vi "HAPS_main_Phase_Cali.vi"() -> ()   [LabVIEW 2023, in "HAPS.lvlib"]
uses:
  HAPS.lvlib
  MCU_Function.ctl
  set_ele.ctl
  HAPS_SerialPort.ctl
  HAPS_MCU_ELE_Func.ctl
panel:
  out "ele_gain":i32
  out "comn_gain":i32
  out "Duration":dbl
  in  "Init?":bool
  out "In-Phase : Phase(degree)":dbl[](graph)
  out "In-Phase : Gain(dB)":dbl[](graph)
  out "channel":i32
  out "chain_id":i32
  out "group":i32
  out "array_id":i32
  in  "Phase diff. Criteria":dbl format="%#_13g"
  in  "Tx/Rx":enum16{"Rx", "Tx"}(ring)=enum."Tx"
  in  "array_id (MCU index)":i32
  in  "MCU_UART_addr":refnum<visa-resource-name>="COM1"
  in  "Max Steps":i32=10
  in  "Target(degree)":dbl format="%#_13g"
  in  "SweepPoints":i32=11
  in  "sParameter":i32=21
  in  "Stop_Freq(GHz)":dbl=39.5
  in  "Start_Freq(GHz)":dbl=38.5
  in  "VISA resource name":refnum<visa-resource-name>="TCPIP0::192.168.119.45::inst0::INSTR"
  in  "HAPS_Equipment":enum16{"Keysight", "R&S"}(ring)=enum."R&S"
  # "TCPIP0::192.168.119.45::inst0::INSTR"
  # "HAPS_24x24_Phase_Calibration"
  # "VNA"
  # "TCPIP0::192.168.1.31::hislip0::INSTR"
  # "Test Status"
  # "DUT"
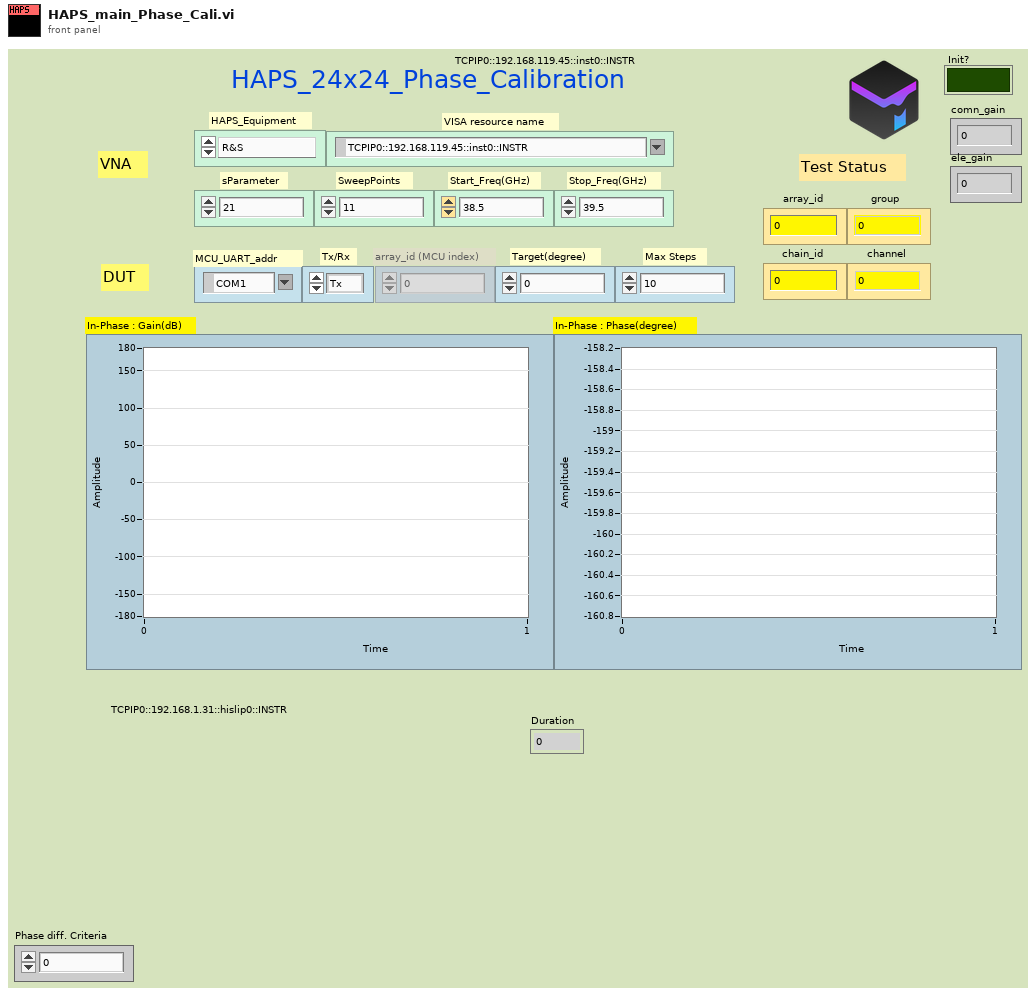
[diagram p1: front panel]
types:
  T1 = typedef "HAPS.lvlib/HAPS_SerialPort.ctl" = enum16{"Init", "Close", "CMD", "Flush"}
  T2 = typedef "HAPS.lvlib/HAPS_MCU_ELE_Func.ctl" = enum16{"array_init", "set_com_gain", "set_ch_gain_phase", "set_pd_range", "get_preamp_temp", "get_bfic_temp", "get_tx_pd", "ch_on", "ch_on_2", "ch_ctrl_all", "array_ctrl_src"}
  T3 = typedef "HAPS.lvlib/set_ele.ctl" = cluster{"ch":i32, "chain_id":i32, "group":i32, "array_id":i32, "ele_phase":i32, "ele_gain":i32, "com_gain":i32, "pd_range":i32}
  T4 = typedef "HAPS.lvlib/MCU_Function.ctl" = cluster{"Tx/Rx":enum16{"Rx", "Tx"}, "Enable?":enum16{"OFF", "On"}, "Source":enum16{"MCU", "ACU"}}
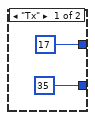
[diagram p2: hidden frame]
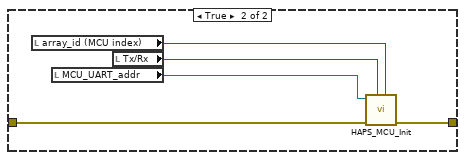
[diagram p3: hidden frame]
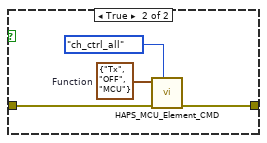
[diagram p4: hidden frame]
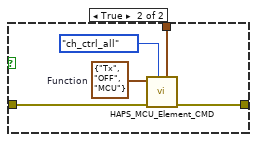
[diagram p6: hidden frame]
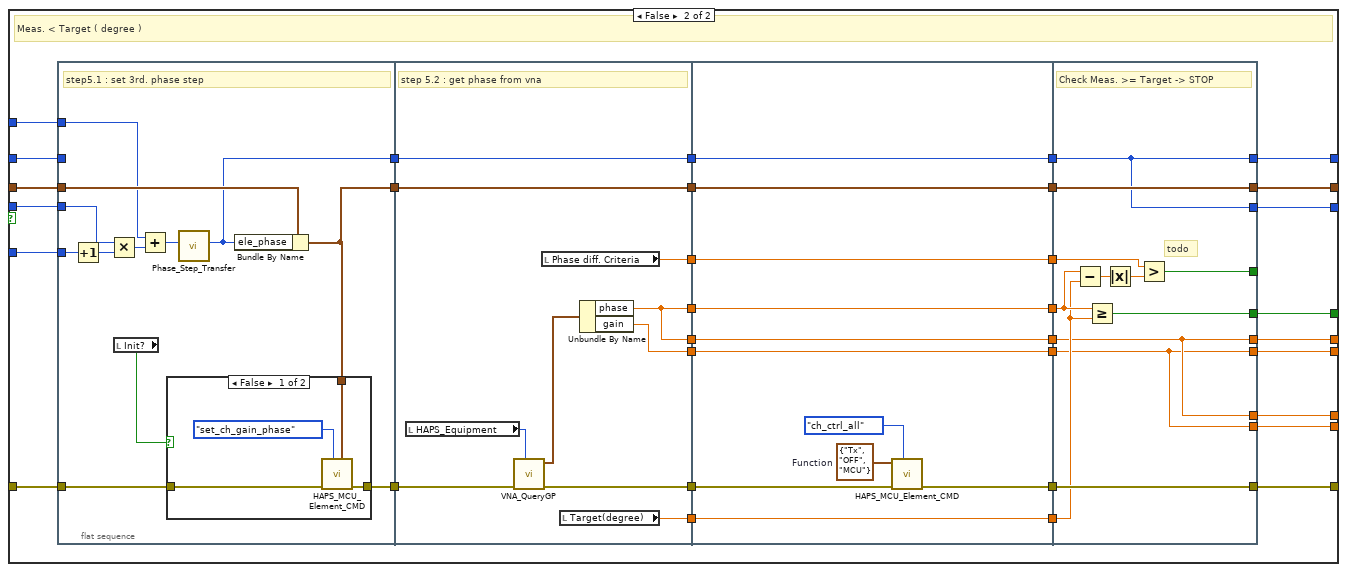
[diagram p10: hidden frame]
diagram:
  n1 = flat-sequence {
    tunnel: [w23] -> w16
    tunnel: [w30] -> w15
    tunnel: [errorcluster {"status"=FALSE, "code"=0, "source"=""} ("error in")] -> w13
    tunnel: ["sParameter"] -> w11
    tunnel: ["VISA resource name"] -> w10
    tunnel: ["Start_Freq(GHz)"] -> w9
    tunnel: ["Stop_Freq(GHz)"] -> w8
    tunnel: ["SweepPoints"] -> w7
    tunnel: ["HAPS_Equipment"] -> w6
    tunnel: [w20] -> w4
    tunnel: w16 -> [w47]
    tunnel: w15 -> [_]
    tunnel: [w47] -> w14
    tunnel: w13 -> [w46]
    tunnel: [w38] -> w12
    tunnel: w11 -> [w45]
    tunnel: w10 -> [w44]
    tunnel: w9 -> [w43]
    tunnel: w8 -> [w42]
    tunnel: w7 -> [w41]
    tunnel: w6 -> [w37]
    tunnel: [w35] -> w5
    tunnel: w4 -> [w35]
    tunnel: w14 -> [w66]
    tunnel: w12 -> [w67]
    tunnel: w5 -> [w63]
    tunnel: [w63] -> w3
    tunnel: [w62] -> w2
    tunnel: [w60] -> w1
    tunnel: [w509] -> _
    tunnel: w3 -> [w509]
    tunnel: w2 -> [w511]
    tunnel: w1 -> [w501]
    frame #0 {
      w21 = dbl[] []
      w23 = T3 {"ch"=0, "chain_id"=0, "group"=0, "array_id"=0, "ele_phase"=0, "ele_gain"=0, "com_gain"=0, "pd_range"=0}  # set_ele
      w30 = T4 {"Tx/Rx"=enum."Tx", "Enable?"=enum."OFF", "Source"=enum."MCU"}  # Function
      # "Init"
      n2 = case shown="\"Rx\"" "Tx/Rx" {
        tunnel: [17 ("comn_ele_gain") 17 ("comn_ele_gain")] -> w18
        tunnel: [35 ("comn_ele_gain") 22 ("comn_ele_gain")] -> w17
        frame "Tx" {
        }
        frame "Rx" {
        }
      }
      "comn_gain" <- w18
      "ele_gain" <- w17
      n3 = Get Date/Time In Seconds() -> (seconds since 1Jan1904=w20:timestamp)
      "In-Phase : Gain(dB)" <- w21
      "In-Phase : Phase(degree)" <- w21
    }
    frame #1 {
      # "settting before Calibration"
      n4 = call "VNA_init.vi"("Stop_Freq(GHz)"=w42, "HAPS_MCU_CMD"=w37, "Start_Freq(GHz)"=w43, "sParameter"=w45, "error in"=w46, "SweepPoints"=w41, "Mark no."=1, "VISA resource name"=w44) -> ("error out"=w39:errorcluster)  [unwired: 3 in]
      n5 = case shown="False" "Init?" {
        tunnel: w39 -> [w54 w59]
        tunnel: [w50 w58] -> w38
        frame False {
          n6 = local read "MCU_UART_addr"() -> (w52:refnum<visa-resource-name>)
          n7 = call "HAPS_MCU_SerialPort.vi"("HAPS_SerialPort_Func"=HAPS_SerialPort."Init", "error in"=w54, "VISA resource name"=w52) -> ("error out"=w51:errorcluster)  [unwired: 6 in, 2 out]
          n8 = call "HAPS_MCU_SerialPort.vi"("Command"="log_en 0", "HAPS_SerialPort_Func"=enum16{"Init", "Close", "CMD"}."CMD" ("HAPS_SerialPort"), "error in"=w51) -> ("error out"=w50:errorcluster)  [unwired: 6 in, 2 out]
        }
        frame True {
          n9 = local read "array_id (MCU index)"() -> (w56:i32)
          n10 = local read "MCU_UART_addr"() -> (w57:refnum<visa-resource-name>)
          n11 = local read "Tx/Rx"() -> (w55:enum16{"Rx", "Tx"})
          n12 = call "HAPS_MCU_Init.vi"("array_id"=w56, "Tx/Rx"=w55, "error in"=w59, "VISA resource name"=w57) -> ("error out"=w58:errorcluster)  [unwired: 7 in]
        }
      }
    }
    frame #2 {
      # "Calibration"
      n13 = for {
        N: 1 -> [_]
        shift-right: [w77] -> _
        shift-left: w66 -> [w73]
        shift-right: [w76] -> w62
        shift-left: string[][] [] -> [w71]
        shift-right: [w75] -> _
        shift-left: w67 -> [w74]
        shift-right: [w68] -> w60
        shift-left: string[][] [] -> [w69]
        i -> [w72]
        w70 = dbl[] []
        # "group ( 0~2 )"
        n14 = for {
          N: 1 -> [_]
          shift-right: [w92] -> w77
          shift-left: w73 -> [w88]
          shift-right: [w91] -> w76
          shift-left: w71 -> [w85]
          shift-right: [w90] -> w75
          shift-left: w74 -> [w89]
          tunnel: w72 -> [w87]
          shift-right: [w82] -> _
          shift-left: w70 -> [w84]
          shift-right: [w81] -> _
          shift-left: w70 -> [w83]
          shift-right: [w79] -> w68
          shift-left: w69 -> [w80]
          i -> [w86]
          # "Chain_id ( 0~11 )"
          n15 = for {
            N: 2 -> [_]
            shift-right: [w164] -> w92
            shift-left: w88 -> [w98]
            shift-right: [w154] -> w91
            shift-left: w85 -> [w155]
            shift-right: [w96] -> w90
            shift-left: w89 -> [w104]
            tunnel: w87 -> [w101]
            tunnel: w86 -> [w100]
            shift-right: [w144] -> w82
            shift-left: w84 -> [w151]
            shift-right: [w143] -> w81
            shift-left: w83 -> [w149]
            shift-right: [w138] -> w79
            shift-left: w80 -> [w142]
            i -> [w99]
            # "Channel ( 0~15 )"
            n16 = local read "array_id (MCU index)"() -> (w102:i32)
            n17 = Bundle By Name(cluster=w98, "array_id"=w102, "group"=w101, "chain_id"=w100, "ch"=w99) -> (w97:T3)
            n18 = call "HAPS_MCU_Element_CMD.vi"("set_ele"=w97, "HAPS_MCU_ELE_Func."=HAPS_MCU_ELE_Func."ch_on", "error in"=w104) -> ("error out"=w103:errorcluster)  [unwired: 7 in, 1 out]
            n19 = flat-sequence {
              tunnel: w97 -> [w188]
              tunnel: w103 -> [w189]
              tunnel: [w190] -> w169
              tunnel: [w186] -> w167
              tunnel: w99 -> [w185]
              tunnel: [w184] -> w156
              tunnel: w155 -> [w184]
              tunnel: w101 -> [w182]
              tunnel: w100 -> [w181]
              tunnel: [w180] -> w152
              tunnel: w151 -> [w180]
              tunnel: [w179] -> w150
              tunnel: w149 -> [w179]
              tunnel: w142 -> [w178]
              tunnel: [w178] -> w141
              tunnel: w169 -> [w206]
              tunnel: [w207] -> w137
              tunnel: [w205] -> w135
              tunnel: [w204] -> w133
              tunnel: w167 -> [w204]
              tunnel: [w201] -> w131
              tunnel: w156 -> [w201]
              tunnel: [w200] -> w129
              tunnel: w152 -> [w200]
              tunnel: [w199] -> w127
              tunnel: w150 -> [w199]
              tunnel: w141 -> [w198]
              tunnel: [w198] -> w125
              tunnel: w137 -> [w213]
              tunnel: [w214] -> w136
              tunnel: w135 -> [w219]
              tunnel: [w219] -> w134
              tunnel: w133 -> [w212]
              tunnel: [w212] -> w132
              tunnel: w131 -> [w218]
              tunnel: [w218] -> w130
              tunnel: w129 -> [w217]
              tunnel: [w217] -> w128
              tunnel: w127 -> [w216]
              tunnel: [w216] -> w126
              tunnel: w125 -> [w215]
              tunnel: [w215] -> w124
              tunnel: w136 -> [w234]
              tunnel: w134 -> [w231]
              tunnel: w132 -> [w233]
              tunnel: [w235] -> w168
              tunnel: [w232] -> w166
              tunnel: [w231] -> w165
              tunnel: [w230] -> w157
              tunnel: w130 -> [w230]
              tunnel: w128 -> [w229]
              tunnel: w126 -> [w228]
              tunnel: [w229] -> w148
              tunnel: [w228] -> w147
              tunnel: w124 -> [w227]
              tunnel: [w227] -> w140
              tunnel: w168 -> [w255]
              tunnel: w166 -> [w247]
              tunnel: [w256] -> w123
              tunnel: [w250] -> w121
              tunnel: [w249] -> w119
              tunnel: [w247] -> w117
              tunnel: [w246] -> w115
              tunnel: w165 -> [w246]
              tunnel: [w244] -> w113
              tunnel: w157 -> [w244]
              tunnel: [w243] -> w111
              tunnel: w148 -> [w243]
              tunnel: [w242] -> w109
              tunnel: w147 -> [w242]
              tunnel: w140 -> [w241]
              tunnel: [w241] -> w107
              tunnel: w123 -> [w258]
              tunnel: [w259] -> w122
              tunnel: w121 -> [w267]
              tunnel: [w267] -> w120
              tunnel: w119 -> [w266]
              tunnel: [w266] -> w118
              tunnel: w117 -> [w265]
              tunnel: [w265] -> w116
              tunnel: w115 -> [w264]
              tunnel: [w264] -> w114
              tunnel: w113 -> [w263]
              tunnel: [w263] -> w112
              tunnel: w111 -> [w262]
              tunnel: [w262] -> w110
              tunnel: w109 -> [w261]
              tunnel: [w261] -> w108
              tunnel: w107 -> [w260]
              tunnel: [w260] -> w106
              tunnel: w122 -> [w285]
              tunnel: w120 -> [w286]
              tunnel: w118 -> [w287]
              tunnel: w116 -> [w288]
              tunnel: w114 -> [w273]
              tunnel: [w284] -> w163
              tunnel: [w283] -> w162
              tunnel: [w282] -> w161
              tunnel: [w281] -> w160
              tunnel: [w280] -> w159
              tunnel: [w279] -> w158
              tunnel: w112 -> [w279]
              tunnel: [w278] -> w153
              tunnel: w110 -> [w277]
              tunnel: w108 -> [w276]
              tunnel: [w277] -> w146
              tunnel: [w276] -> w145
              tunnel: w106 -> [w275]
              tunnel: [w274] -> w139
              tunnel: [w500] -> w164
              tunnel: w163 -> [w500]
              tunnel: w162 -> [w499]
              tunnel: w161 -> [w471]
              tunnel: w160 -> [w472]
              tunnel: w159 -> [w494]
              tunnel: w158 -> [w478]
              tunnel: [w480] -> w154
              tunnel: [w479] -> w95
              tunnel: w153 -> [w479]
              tunnel: w146 -> [w475]
              tunnel: w145 -> [w474]
              tunnel: [w477] -> w144
              tunnel: [w476] -> w143
              tunnel: w139 -> [w470]
              tunnel: [w470] -> w138
              frame #0 {
                w191 = 0  # pd_range
                w192 = 0  # Init_Phase_Step
                # "step 1. : First get phase step \"0\" for element BFIC"
                n20 = local read "array_id (MCU index)"() -> (w183:i32)
                "array_id" <- w183
                n21 = local read "ele_gain"() -> (w175:i32)
                n22 = local read "comn_gain"() -> (w176:i32)
                n23 = Bundle By Name(cluster=w188, "array_id"=w183, "group"=w182, "chain_id"=w181, "ch"=w185, "com_gain"=w176, "ele_gain"=w175, "ele_phase"=w192, "pd_range"=w191) -> (w186:T3)
                n24 = case shown="False" FALSE {
                  tunnel: [w196 w197] -> w190
                  tunnel: w189 -> [w195 w197]
                  tunnel: HAPS_MCU_ELE_Func."set_ch_gain_phase" ("HAPS_MCU_ELE_Func.") -> [w194 _]
                  tunnel: w186 -> [w193 _]
                  frame False {
                    n25 = call "HAPS_MCU_Element_CMD.vi"("set_ele"=w193, "HAPS_MCU_ELE_Func."=w194, "error in"=w195) -> ("error out"=w196:errorcluster)  [unwired: 7 in, 1 out]
                  }
                  frame True {
                  }
                }
                "group" <- w182
                "chain_id" <- w181
                "channel" <- w185
              }
              frame #1 {
                # "todo:gain"
                # "step 2. : get first pahse data from vna"
                n26 = local read "HAPS_Equipment"() -> (w202:enum16{"Keysight", "R&S"})
                n27 = call "VNA_QueryGP.vi"("HAPS_Equipment"=w202, "error in"=w206) -> ("error out"=w207:errorcluster, "queryMarker"=w208:cluster{"gain":dbl, "phase":dbl})  [unwired: 8 in]
                n28 = Unbundle By Name(w204) -> ("ele_phase"=w203:i32)
                n29 = local read "Target(degree)"() -> (w210:dbl)
                n30 = Unbundle By Name(w208) -> ("phase"=w209:dbl)  [unwired: 1 out]
                n31 = call "Estimation_Steps.vi"("Target(degree)"=w210, "Source_Phase_Step"=w203, "Input_Phase(degree)"=w209) -> ("Esitmation_Step"=w205:i32)  [unwired: 7 in, 1 out]
              }
              frame #2 {
                n32 = case shown="False" FALSE {
                  tunnel: [w220 w225] -> w214
                  tunnel: w213 -> [w220 w224]
                  tunnel: w212 -> [_ w222]
                  frame False {
                  }
                  frame True {
                    w221 = T4 {"Tx/Rx"=enum."Tx", "Enable?"=enum."OFF", "Source"=enum."MCU"}  # Function
                    n33 = call "HAPS_MCU_Element_CMD.vi"("set_ele"=w222, "HAPS_MCU_ELE_Func."=HAPS_MCU_ELE_Func."ch_ctrl_all", "error in"=w224, "Function"=w221) -> ("error out"=w225:errorcluster)  [unwired: 6 in, 1 out]
                  }
                }
              }
              frame #3 {
                # "source.\nphase step"
                # "step 3.  set estimation phase step in second time"
                n34 = Bundle By Name(cluster=w233, "ele_phase"=w231) -> (w232:T3)
                n35 = case shown="False" FALSE {
                  tunnel: [w239 w240] -> w235
                  tunnel: w234 -> [w238 w240]
                  tunnel: w232 -> [w237 _]
                  frame False {
                    n36 = call "HAPS_MCU_Element_CMD.vi"("set_ele"=w237, "HAPS_MCU_ELE_Func."=HAPS_MCU_ELE_Func."set_ch_gain_phase", "error in"=w238) -> ("error out"=w239:errorcluster)  [unwired: 7 in, 1 out]
                  }
                  frame True {
                  }
                }
              }
              frame #4 {
                # "todo:gain"
                # "step 4. : get second time pahse from vna"
                n37 = local read "HAPS_Equipment"() -> (w245:enum16{"Keysight", "R&S"})
                n38 = call "VNA_QueryGP.vi"("HAPS_Equipment"=w245, "error in"=w255) -> ("error out"=w256:errorcluster, "queryMarker"=w251:cluster{"gain":dbl, "phase":dbl})  [unwired: 8 in]
                n39 = Unbundle By Name(w251) -> ("phase"=w248:dbl)  [unwired: 1 out]
                n40 = local read "Target(degree)"() -> (w252:dbl)
                n41 = Greater Or Equal?(x=w248, y=w252) -> (x >= y?=w250:bool)
                n42 = Select(t=1, s=w250, f=-1) -> (s? t:f=w249:i32)
              }
              frame #5 {
                n43 = local read "Init?"() -> (w257:bool)
                n44 = case shown="False" w257 {
                  tunnel: [w269 w272] -> w259
                  tunnel: w258 -> [w268 w272]
                  frame False {
                    w271 = T4 {"Tx/Rx"=enum."Tx", "Enable?"=enum."OFF", "Source"=enum."MCU"}  # Function
                    n45 = call "HAPS_MCU_Element_CMD.vi"("HAPS_MCU_ELE_Func."=HAPS_MCU_ELE_Func."ch_ctrl_all", "error in"=w268, "Function"=w271) -> ("error out"=w269:errorcluster)  [unwired: 7 in, 1 out]
                  }
                  frame True {
                  }
                }
              }
              frame #6 {
                # "source.\nphase step"
                # "Mea. >= Target"
                # "source.\ndegree"
                # "step 5. : find in-phase step"
                n46 = for {
                  N: "Max Steps" -> [_]
                  shift-right: [w313] -> w284
                  shift-left: w288 -> [w316]
                  shift-right: [w314] -> w278
                  shift-left: w285 -> [w319]
                  shift-right: [w307] -> w280
                  shift-left: w273 -> [w315]
                  tunnel: w286 -> [w320]
                  tunnel: w287 -> [w317]
                  shift-right: [w312] -> w283
                  shift-left: _ -> [_]
                  shift-right: [w298] -> w281
                  shift-left: _ -> [_]
                  shift-right: [w297] -> w282
                  shift-left: _ -> [_]
                  shift-right: [w291] -> w274
                  shift-left: w275 -> [w293]
                  tunnel: w273 -> [w290]
                  i -> [w318]
                  stop <- w312 stop-if-true
                  n47 = case shown="True" w320 {
                    tunnel: w319 -> [w346 w419]
                    tunnel: w318 -> [w345 w418]
                    tunnel: w317 -> [w344 w417]
                    tunnel: w316 -> [w343 w416]
                    tunnel: w315 -> [w342 w415]
                    tunnel: [w341 w414] -> w314
                    tunnel: [w340 w413] -> w313
                    tunnel: [w339 w412] -> w307
                    tunnel: [w331 w408] -> w312
                    tunnel: [w330 w407] -> _
                    tunnel: [w327 w406] -> w298
                    tunnel: [w326 w405] -> w297
                    tunnel: [w323 w404] -> _
                    tunnel: [w322 w403] -> _
                    tunnel: w290 -> [w321 w402]
                    frame True {
                      # "Meas. >= Target ( degree )"
                      n48 = flat-sequence {
                        tunnel: w346 -> [w355]
                        tunnel: w345 -> [w358]
                        tunnel: w344 -> [w357]
                        tunnel: w343 -> [w352]
                        tunnel: w342 -> [_]
                        tunnel: [w356] -> w338
                        tunnel: [w353] -> w337
                        tunnel: [w349] -> w336
                        tunnel: w321 -> [w347]
                        tunnel: w338 -> [w370]
                        tunnel: w337 -> [w373]
                        tunnel: w336 -> [w372]
                        tunnel: [w371] -> w335
                        tunnel: [w373] -> w334
                        tunnel: [w372] -> w333
                        tunnel: [w367] -> w332
                        tunnel: [w368] -> w329
                        tunnel: [w364] -> w328
                        tunnel: [w366] -> w325
                        tunnel: [w367] -> w324
                        tunnel: [w383] -> w331
                        tunnel: [w382] -> w339
                        tunnel: [w384] -> w340
                        tunnel: [w385] -> w341
                        tunnel: w335 -> [w385]
                        tunnel: w334 -> [w384]
                        tunnel: w333 -> [w382]
                        tunnel: w332 -> [w381]
                        tunnel: [w382] -> w330
                        tunnel: w329 -> [w379]
                        tunnel: w328 -> [w377]
                        tunnel: [w376] -> _
                        tunnel: [w375] -> w327
                        tunnel: [w374] -> w326
                        tunnel: w325 -> [w374]
                        tunnel: w324 -> [w375]
                        tunnel: [w375] -> w323
                        tunnel: [w374] -> w322
                        frame #0 {
                          # "step5.1 : set 3rd. phase step"
                          n49 = Increment(x=w358) -> (x+1=w354:i32)
                          n50 = local read "Init?"() -> (w348:bool)
                          n51 = Multiply(x=w357, y=w354) -> (x*y=w351:i32)
                          n52 = Add(x=w347, y=w351) -> (x+y=w350:i32)
                          n53 = call "Phase_Step_Transfer.vi"("Input_Phase_Step"=w350) -> ("Output_Phase_Step"=w349:i32)  [unwired: 10 in]
                          n54 = Bundle By Name(cluster=w352, "ele_phase"=w349) -> (w353:T3)
                          n55 = case shown="False" w348 {
                            tunnel: [w362 w363] -> w356
                            tunnel: w355 -> [w361 w363]
                            tunnel: w353 -> [w360 _]
                            frame False {
                              n56 = call "HAPS_MCU_Element_CMD.vi"("set_ele"=w360, "HAPS_MCU_ELE_Func."=HAPS_MCU_ELE_Func."set_ch_gain_phase", "error in"=w361) -> ("error out"=w362:errorcluster)  [unwired: 7 in, 1 out]
                            }
                            frame True {
                            }
                          }
                        }
                        frame #1 {
                          # "step 5.2 : get phase from vna"
                          n57 = local read "HAPS_Equipment"() -> (w365:enum16{"Keysight", "R&S"})
                          n58 = call "VNA_QueryGP.vi"("HAPS_Equipment"=w365, "error in"=w370) -> ("error out"=w371:errorcluster, "queryMarker"=w369:cluster{"gain":dbl, "phase":dbl})  [unwired: 8 in]
                          n59 = local read "Phase diff. Criteria"() -> (w364:dbl)
                          n60 = local read "Target(degree)"() -> (w368:dbl)
                          n61 = Unbundle By Name(w369) -> ("phase"=w367:dbl, "gain"=w366:dbl)
                        }
                        frame #2 {
                          # "todo"
                          # "Check Meas. <= Target => STOP"
                          n62 = Subtract(x=w381, y=w379) -> (x-y=w380:dbl)
                          n63 = Less Or Equal?(x=w381, y=w379) -> (x <= y?=w383:bool)
                          n64 = Absolute Value(x=w380) -> (abs(x)=w378:dbl)
                          n65 = Greater?(x=w377, y=w378) -> (0:w376:bool)
                        }
                      }
                    }
                    frame False {
                      # "Meas. < Target ( degree )"
                      n66 = flat-sequence {
                        tunnel: w419 -> [w428]
                        tunnel: w418 -> [w431]
                        tunnel: w417 -> [w430]
                        tunnel: w416 -> [w425]
                        tunnel: w415 -> [_]
                        tunnel: [w429] -> w411
                        tunnel: [w426] -> w410
                        tunnel: [w422] -> w409
                        tunnel: w402 -> [w420]
                        tunnel: w411 -> [w443]
                        tunnel: w410 -> [w446]
                        tunnel: w409 -> [w445]
                        tunnel: [w444] -> w401
                        tunnel: [w446] -> w399
                        tunnel: [w445] -> w397
                        tunnel: [w440] -> w395
                        tunnel: [w441] -> w393
                        tunnel: [w437] -> w391
                        tunnel: [w439] -> w389
                        tunnel: [w440] -> w387
                        tunnel: w401 -> [w447]
                        tunnel: [w448] -> w400
                        tunnel: w399 -> [w457]
                        tunnel: [w457] -> w398
                        tunnel: w397 -> [w456]
                        tunnel: [w456] -> w396
                        tunnel: w395 -> [w455]
                        tunnel: [w455] -> w394
                        tunnel: w393 -> [w454]
                        tunnel: [w454] -> w392
                        tunnel: w391 -> [w453]
                        tunnel: [w453] -> w390
                        tunnel: w389 -> [w452]
                        tunnel: [w452] -> w388
                        tunnel: w387 -> [w451]
                        tunnel: [w451] -> w386
                        tunnel: [w467] -> w408
                        tunnel: [w466] -> w412
                        tunnel: [w468] -> w413
                        tunnel: [w469] -> w414
                        tunnel: w400 -> [w469]
                        tunnel: w398 -> [w468]
                        tunnel: w396 -> [w466]
                        tunnel: w394 -> [w465]
                        tunnel: [w466] -> w407
                        tunnel: w392 -> [w463]
                        tunnel: w390 -> [w461]
                        tunnel: [w460] -> _
                        tunnel: [w459] -> w406
                        tunnel: [w458] -> w405
                        tunnel: w388 -> [w458]
                        tunnel: w386 -> [w459]
                        tunnel: [w459] -> w404
                        tunnel: [w458] -> w403
                        frame #0 {
                          # "step5.1 : set 3rd. phase step"
                          n67 = Increment(x=w431) -> (x+1=w427:i32)
                          n68 = Multiply(x=w430, y=w427) -> (x*y=w424:i32)
                          n69 = local read "Init?"() -> (w421:bool)
                          n70 = Add(x=w420, y=w424) -> (x+y=w423:i32)
                          n71 = call "Phase_Step_Transfer.vi"("Input_Phase_Step"=w423) -> ("Output_Phase_Step"=w422:i32)  [unwired: 10 in]
                          n72 = Bundle By Name(cluster=w425, "ele_phase"=w422) -> (w426:T3)
                          n73 = case shown="False" w421 {
                            tunnel: [w435 w436] -> w429
                            tunnel: w428 -> [w434 w436]
                            tunnel: w426 -> [w433 _]
                            frame False {
                              n74 = call "HAPS_MCU_Element_CMD.vi"("set_ele"=w433, "HAPS_MCU_ELE_Func."=HAPS_MCU_ELE_Func."set_ch_gain_phase", "error in"=w434) -> ("error out"=w435:errorcluster)  [unwired: 7 in, 1 out]
                            }
                            frame True {
                            }
                          }
                        }
                        frame #1 {
                          # "step 5.2 : get phase from vna"
                          n75 = local read "HAPS_Equipment"() -> (w438:enum16{"Keysight", "R&S"})
                          n76 = call "VNA_QueryGP.vi"("HAPS_Equipment"=w438, "error in"=w443) -> ("error out"=w444:errorcluster, "queryMarker"=w442:cluster{"gain":dbl, "phase":dbl})  [unwired: 8 in]
                          n77 = local read "Phase diff. Criteria"() -> (w437:dbl)
                          n78 = local read "Target(degree)"() -> (w441:dbl)
                          n79 = Unbundle By Name(w442) -> ("phase"=w440:dbl, "gain"=w439:dbl)
                        }
                        frame #2 {
                          w449 = T4 {"Tx/Rx"=enum."Tx", "Enable?"=enum."OFF", "Source"=enum."MCU"}  # Function
                          n80 = call "HAPS_MCU_Element_CMD.vi"("HAPS_MCU_ELE_Func."=HAPS_MCU_ELE_Func."ch_ctrl_all", "error in"=w447, "Function"=w449) -> ("error out"=w448:errorcluster)  [unwired: 7 in, 1 out]
                        }
                        frame #3 {
                          # "todo"
                          # "Check Meas. >= Target -> STOP"
                          n81 = Subtract(x=w465, y=w463) -> (x-y=w464:dbl)
                          n82 = Greater Or Equal?(x=w465, y=w463) -> (x >= y?=w467:bool)
                          n83 = Absolute Value(x=w464) -> (abs(x)=w462:dbl)
                          n84 = Greater?(x=w461, y=w462) -> (0:w460:bool)
                        }
                      }
                    }
                  }
                  n85 = property on="Tx/Rx" class="Enum (strict)"() -> ("RingText.Text"=w306:string)  [unwired: 2 in, 2 out]
                  n86 = local read "chain_id"() -> (w310:i32)
                  n87 = local read "array_id"() -> (w308:i32)
                  n88 = local read "channel"() -> (w311:i32)
                  n89 = local read "group"() -> (w309:i32)
                  n90 = Number To Decimal String(number=w308) -> (decimal integer string=w305:string)  [unwired: 1 in]
                  n91 = Number To Decimal String(number=w309) -> (decimal integer string=w304:string)  [unwired: 1 in]
                  n92 = Number To Decimal String(number=w310) -> (decimal integer string=w303:string)  [unwired: 1 in]
                  n93 = Number To Decimal String(number=w311) -> (decimal integer string=w302:string)  [unwired: 1 in]
                  n94 = Number To Decimal String(number=w307) -> (decimal integer string=w301:string)  [unwired: 1 in]
                  n95 = Number To Fractional String(number=w298, precision (6)=i16 3) -> (F-format string=w296:string)  [unwired: 2 in]
                  n96 = Number To Fractional String(number=w297, precision (6)=i16 3) -> (F-format string=w295:string)  [unwired: 2 in]
                  n97 = Build Array(w306, w305, w304, w303, w302, w301, w296, w295, "log") -> (w292:string[])
                  n98 = Build Array (concatenate)(w293, w292) -> (w291:string[][])
                }
              }
              frame #7 {
                # "Result Update"
                n99 = property on="Tx/Rx" class="Enum (strict)"() -> ("RingText.Text"=w487:string)  [unwired: 2 in, 2 out]
                n100 = local read "chain_id"() -> (w496:i32)
                n101 = local read "array_id"() -> (w498:i32)
                n102 = local read "channel"() -> (w495:i32)
                n103 = local read "group"() -> (w497:i32)
                n104 = Build Array (concatenate)(w475, w471) -> (w477:dbl[])
                n105 = Build Array (concatenate)(w474, w472) -> (w476:dbl[])
                n106 = Select(t="Pass", s=w499, f="Failure") -> (s? t:f=w481:string)
                n107 = local write "In-Phase : Phase(degree)"(w476) -> ()
                n108 = local write "In-Phase : Gain(dB)"(w477) -> ()
                n109 = Number To Fractional String(number=w472, precision (6)=i16 3) -> (F-format string=w483:string)  [unwired: 2 in]
                n110 = Number To Decimal String(number=w498) -> (decimal integer string=w489:string)  [unwired: 1 in]
                n111 = Number To Decimal String(number=w497) -> (decimal integer string=w488:string)  [unwired: 1 in]
                n112 = Number To Decimal String(number=w496) -> (decimal integer string=w486:string)  [unwired: 1 in]
                n113 = Number To Decimal String(number=w495) -> (decimal integer string=w485:string)  [unwired: 1 in]
                n114 = Number To Decimal String(number=w494) -> (decimal integer string=w484:string)  [unwired: 1 in]
                n115 = Number To Fractional String(number=w471, precision (6)=i16 3) -> (F-format string=w482:string)  [unwired: 2 in]
                n116 = Build Array(w487, w489, w488, w486, w485, w484, w483, w482, w481) -> (w473:string[])
                n117 = Build Array (concatenate)(w478, w473) -> (w480:string[][])
              }
            }
            n118 = case shown="False" TRUE {
              tunnel: [w170 w172] -> w96
              tunnel: w95 -> [w170 w171]
              frame False {
              }
              frame True {
                w173 = T4 {"Tx/Rx"=enum."Tx", "Enable?"=enum."OFF", "Source"=enum."MCU"}  # Function
                n119 = call "HAPS_MCU_Element_CMD.vi"("HAPS_MCU_ELE_Func."=HAPS_MCU_ELE_Func."ch_ctrl_all", "error in"=w171, "Function"=w173) -> ("error out"=w172:errorcluster)  [unwired: 7 in, 1 out]
              }
            }
          }
        }
      }
    }
    frame #3 {
      n120 = Get Date/Time In Seconds() -> (seconds since 1Jan1904=w510:timestamp)
      n121 = Subtract(x=w510, y=w509) -> (x-y=→"Duration":dbl)
      n122 = local read "array_id"() -> (w505:i32)
      n123 = property on="Tx/Rx" class="Enum (strict)"() -> ("RingText.Text"=w506:string)  [unwired: 2 in, 2 out]
      n124 = local read "array_id"() -> (w514:i32)
      n125 = property on="MCU_UART_addr" class="VISAName"() -> ("Text.Text"=w503:string)  [unwired: 2 in, 2 out]
      n126 = Number To Decimal String(number=w505) -> (decimal integer string=w504:string)  [unwired: 1 in]
      n127 = property on="Tx/Rx" class="Enum (strict)"() -> ("RingText.Text"=w513:string)  [unwired: 2 in, 2 out]
      n128 = property on="MCU_UART_addr" class="VISAName"() -> ("Text.Text"=w517:string)  [unwired: 2 in, 2 out]
      n129 = Number To Decimal String(number=w514) -> (decimal integer string=w515:string)  [unwired: 1 in]
      n130 = Format Into String(format string="HAPS_Phase_Cali_%s_MCU%s_%s_DetailALL", w506, w504, w503) -> (resulting string=w502:string)  [unwired: 2 in, 1 out]
      n131 = Format Into String(format string="HAPS_Phase_Cali_%s_MCU%s_%s", w513, w515, w517) -> (resulting string=w516:string)  [unwired: 2 in, 1 out]
      n132 = call "_save_csv_HAPS_MCU_PhaseCali.vi"("NoteName"=w502, "array in"=w501) -> ()  [unwired: 9 in, 1 out]
      n133 = call "_save_csv_HAPS_MCU_PhaseCali.vi"("NoteName"=w516, "array in"=w511) -> ()  [unwired: 9 in, 1 out]
    }
  }
